vi "Initialize PDM Acquisition.vi"(9 "ProtocolCaptureResourceName":string, 10 "MeasurementConfiguration":T1={"BandStart"=20.0, "BandStop"=20000.0, "Amplitude"=1.0, "Frequency"=1000.0, "FullScaleRange"=2.825, "DataLine"=0, "SampleRate"=12288000, "MeasurementDuration"=19200.0, "Channel"=0, "FrameSyncEdgeForChannel_0"=0, "ChannelCountPerFrame"=2, "ChannelLength"=32, "BitDepth"=24, "Channel_0_offset"=1, "Endianness"=0, "DataJustification"=0, "FrameSyncPulseWidth"=32, "BitClockEdgeSync"=1, "ClockRate"=0, "FrameLength"=0, "NumberOfWords"=0, "Sensitivity"=0.0}) -> (2 "error out":errorcluster, 3 "ObjRefOut":u32)   [LabVIEW 2021]
uses:
  <vilib>/PDM Acquisition Toolkit/host/Classes/Tasks/PCM Input/Controls/DVR PCM Input Task.ctl
  <vilib>/PDM Acquisition Toolkit/host/Classes/Tasks/PCM Input/PCM Input Task.lvclass
  Measurement Configuration.ctl
  <vilib>/PDM Acquisition Toolkit/host/Classes/Tasks/PDM Tasks/Controls/Acquisition Mode.ctl
  <vilib>/PDM Acquisition Toolkit/host/Classes/Session/Controls/Logic Levels.ctl
  <vilib>/PDM Acquisition Toolkit/shared/controls/PCM Data Format Configuration.ctl
  <vilib>/PDM Acquisition Toolkit/shared/controls/Digital Edge.ctl
  <vilib>/PDM Acquisition Toolkit/shared/controls/PCM Bit Endianness.ctl
  <vilib>/PDM Acquisition Toolkit/shared/controls/PCM Data Justification.ctl
  <vilib>/PDM Acquisition Toolkit/shared/controls/PCM Frame Sync Control.ctl
  <vilib>/PDM Acquisition Toolkit/host/API/Public/Create Tasks/Create PCM Input Task.vi
  <vilib>/PDM Acquisition Toolkit/host/API/Public/Configure/Timing/Configure Timing - PCM Input Slave.vi
  <vilib>/PDM Acquisition Toolkit/host/API/Public/Configure/PDM Channel/Configure Microphone Sensitivity FSPA - PCM Input Task.vi
  <vilib>/PDM Acquisition Toolkit/host/API/PDM Acquisition Toolkit.lvlib
  <vilib>/PDM Acquisition Toolkit/host/Classes/Tasks/PDM Tasks/PDM Task.lvclass
  <vilib>/PDM Acquisition Toolkit/host/Classes/Session/DecoderSession.lvclass
  <vilib>/PDM Acquisition Toolkit/shared/PDM Shared.lvlib
panel:
  out "PCM input task out":T2
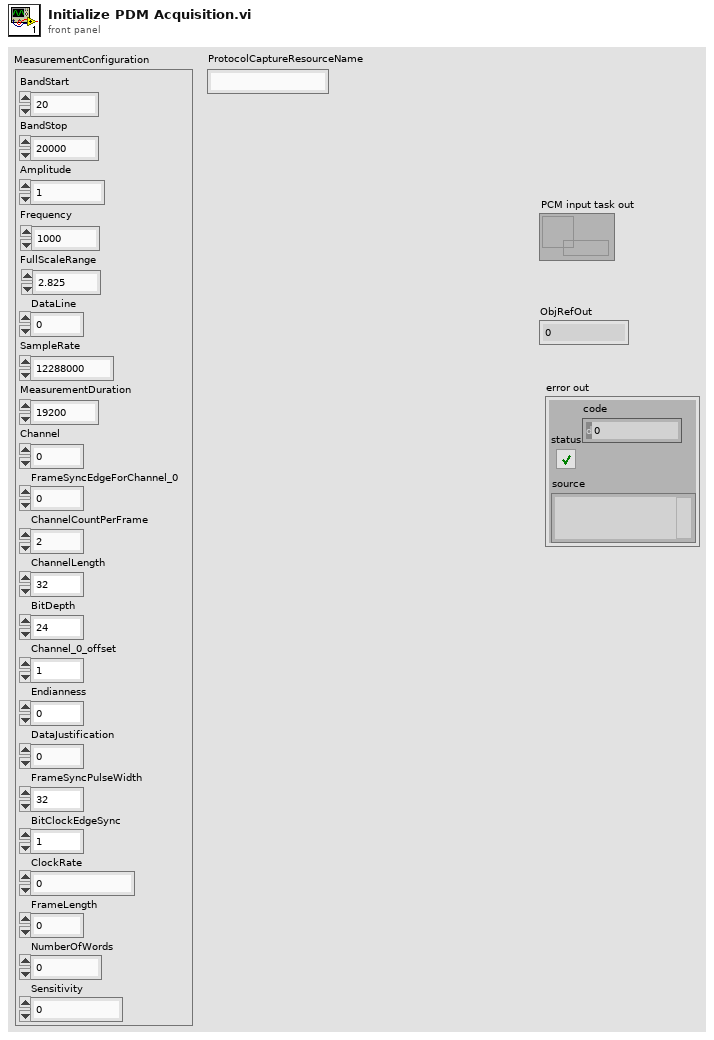
[diagram p1: front panel]
types:
  T1 = typedef "Measurement Configuration.ctl" = cluster{"BandStart":dbl, "BandStop":dbl, "Amplitude":dbl, "Frequency":dbl, "FullScaleRange":dbl, "DataLine":u32, "SampleRate":u32, "MeasurementDuration":dbl, "Channel":u32, "FrameSyncEdgeForChannel_0":u32, "ChannelCountPerFrame":u32, "ChannelLength":u32, "BitDepth":u32, "Channel_0_offset":u32, "Endianness":u32, "DataJustification":u32, "FrameSyncPulseWidth":u32, "BitClockEdgeSync":u32, "ClockRate":u32, "FrameLength":u32, "NumberOfWords":u32, "Sensitivity":dbl}
  T2 = typedef "PDM Acquisition Class Library.lvlib/PCM Input Task.lvclass/DVR PCM Input Task.ctl" = refnum<data-value>
  T3 = typedef "PDM Shared.lvlib/PCM Frame Sync Control.ctl" = cluster{"Frame Length":u16, "Frame Sync Pulse Width":u16, "Bit Clock Edge  Sync":T4}
  T4 = typedef "PDM Shared.lvlib/Digital Edge.ctl" = enum8{"Rising", "Falling"}
  T5 = typedef "PDM Shared.lvlib/PCM Data Format Configuration.ctl" = cluster{"Frame Sync Edge for Channel 0":T4, "Channel Count Per Frame":u8, "Channel Length":u16, "Bit Depth":u8, "Channel 0 Offset":u16, "Endianness":T6, "Data Justification":T7}
  T6 = typedef "PDM Shared.lvlib/PCM Bit Endianness.ctl" = enum16{"MSB First", "LSB First"}
  T7 = typedef "PDM Shared.lvlib/PCM Data Justification.ctl" = enum16{"Left Justified", "Right Justified"}
  T8 = typedef "PDM Acquisition Class Library.lvlib/DecoderSession.lvclass/Logic Levels.ctl" = enum16{"3.3 V", "1.8 V", "1.2 V"}
  T9 = typedef "PDM Acquisition Class Library.lvlib/PDM Task.lvclass/Acquisition Mode.ctl" = enum16{"Finite", "Continuous"}
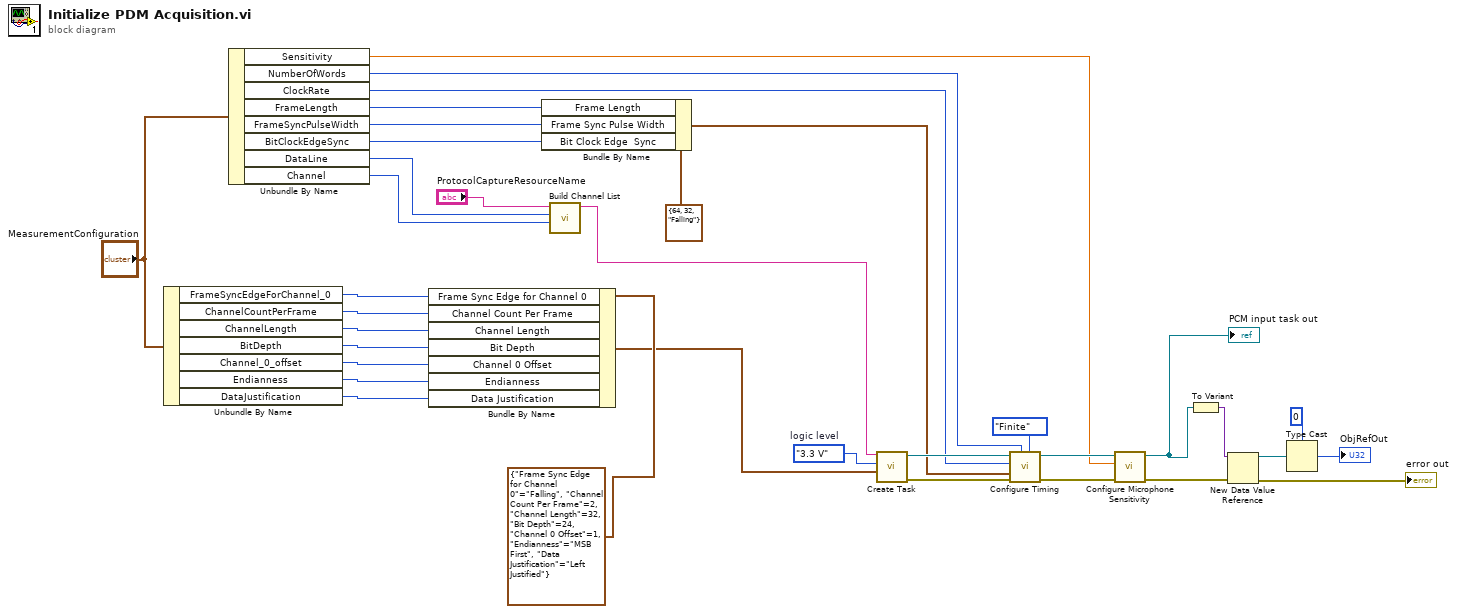
[diagram p0: block diagram]
diagram:
  w32 = Logic_Levels."3.3 V"  # logic level
  n1 = Unbundle By Name("MeasurementConfiguration") -> ("FrameSyncEdgeForChannel_0"=w7:u32, "ChannelCountPerFrame"=w6:u32, "ChannelLength"=w5:u32, "BitDepth"=w4:u32, "Channel_0_offset"=w3:u32, "Endianness"=w2:u32, "DataJustification"=w1:u32)
  n2 = Unbundle By Name("MeasurementConfiguration") -> ("Sensitivity"=w14:dbl, "NumberOfWords"=w13:u32, "ClockRate"=w12:u32, "FrameLength"=w21:u32, "FrameSyncPulseWidth"=w20:u32, "BitClockEdgeSync"=w19:u32, "DataLine"=w18:u32, "Channel"=w17:u32)
  n3 = Bundle By Name(cluster=T5 {"Frame Sync Edge for Channel 0"=enum."Falling", "Channel Count Per Frame"=2, "Channel Length"=32, "Bit Depth"=24, "Channel 0 Offset"=1, "Endianness"=enum."MSB First", "Data Justification"=enum."Left Justified"} ("PCM data configuration"), "Frame Sync Edge for Channel 0"=w7, "Channel Count Per Frame"=w6, "Channel Length"=w5, "Bit Depth"=w4, "Channel 0 Offset"=w3, "Endianness"=w2, "Data Justification"=w1) -> (w8:T5)
  n4 = Bundle By Name(cluster=T3 {"Frame Length"=64, "Frame Sync Pulse Width"=32, "Bit Clock Edge  Sync"=enum."Falling"} ("Frame Sync Clock Control"), "Frame Length"=w21, "Frame Sync Pulse Width"=w20, "Bit Clock Edge  Sync"=w19) -> (w30:T3)
  n5 = call "Build Channel List.vi"("Channel"=w17, "Data line"=w18, "Protocol capture resource name"="ProtocolCaptureResourceName") -> ("String"=w27:string)  [unwired: 8 in]
  n6 = call-poly <vilib>:"Create Task.vi"("PCM data configuration"=w8, "logic level"=w32, "channel list"=w27) -> ("error out"=w34:errorcluster, "PCM input task out"=w35:T2)  [unwired: 7 in]
  n7 = call-poly <vilib>:"Configure Timing.vi"("acquisition mode"=Acquisition_Mode."Finite", "Frame Sync Clock Control"=w30, "number of words per channel"=w13, "error in"=w34, "Bit Clock rate"=w12, "PCM input task in"=w35) -> ("error out"=w28:errorcluster, "PCM input task out"=w29:T2)  [unwired: 4 in]
  n8 = call-poly <vilib>:"Configure Microphone Sensitivity.vi"("error in"=w28, "microphone sensitivity (FS/Pa)"=w14, "PCM input task in"=w29) -> ("error out"=w23:errorcluster, "PCM input task out"=w15:T2)  [unwired: 7 in]
  "PCM input task out" <- w15
  n9 = To Variant(anything=w15) -> (Variant=w25:variant)
  n10 = New Data Value Reference(data value=w25, error in=w23) -> (data value reference=w26:refnum<data-value>, error out=→"error out":errorcluster)
  n11 = Type Cast(type=u32 0, x=w26) -> (*(type *) &x=→"ObjRefOut":u32)
